vi "Configure Session.vi"(8 "error in":errorcluster, 11 "Plugin in":refnum<class "Power Spectrum Density.lvclass">) -> (0 "error out":errorcluster, 3 "Plugin out":refnum<class "Power Spectrum Density.lvclass">)   [LabVIEW 2023, in "Power Spectrum Density.lvlib" / "Power Spectrum Density.lvclass"]
uses:
  Power Spectrum Density.lvclass
  C:/Program Files/National Instruments/LabVIEW 2023/vi.lib/FlexLogger/SDK/PluginSDK.lvlibp/PEFClasses/SDK/Plugin/Plugin.lvclass
  Power Spectrum Density Data.ctl
  <vilib>/measure/maspectr.llb/Power Spectrum and PSD Export Mode.ctl
  <vilib>/Analysis/4window.llb/windowTd.ctl
  <vilib>/FlexLogger/SDK/PluginSDK.lvlibp/PEFClasses/SDK/Processing Element/Timing Parameters.ctl
  <vilib>/FlexLogger/SDK/PluginSDK.lvlibp/PEFClasses/SDK/Processing Element/Timing Method.ctl
  <vilib>/FlexLogger/SDK/PluginSDK.lvlibp/PEFClasses/SDK/System Interface/Resampling Mode.ctl
  Buffer Manager Function.ctl
  Power Spectrum Density.lvclass/Power Spectrum Density.ctl
  Power Spectrum Density Global.vi
  <vilib>/FlexLogger/SDK/PluginSDK.lvlibp/PEFClasses/SDK/Plugin/ParameterAccess/Read Enum.vi
  <vilib>/FlexLogger/SDK/PluginSDK.lvlibp/PEFClasses/SDK/Plugin/ParameterAccess/Read Boolean.vi
  <vilib>/FlexLogger/SDK/PluginSDK.lvlibp/PEFClasses/SDK/Plugin/ParameterAccess/Read I32.vi
  <vilib>/FlexLogger/SDK/PluginSDK.lvlibp/PEFClasses/SDK/Plugin/ParameterAccess/Read DBL.vi
  <vilib>/FlexLogger/SDK/PluginSDK.lvlibp/PEFClasses/SDK/Plugin/Plugin.lvclass
  <vilib>/Utility/LVLibp/NI_PackedLibraryUtility.lvlib
  <vilib>/measure/NI_MAPro.lvlib
  <vilib>/Analysis/NI_AALPro.lvlib
  <vilib>/FlexLogger/SDK/PluginSDK.lvlibp/PEFClasses/SDK/Processing Element/Processing Element.lvclass
  <vilib>/FlexLogger/SDK/PluginSDK.lvlibp/PEFClasses/SDK/System Interface/System Interface.lvclass
  C:/Program Files/National Instruments/LabVIEW 2023/vi.lib/FlexLogger/SDK/PluginSDK.lvlibp/PEFClasses/SDK/Processing Element/Processing Element.lvclass
  C:/Users/Administrator/Documents/LabVIEW Projects/FlexLogger IO Plug-ins/Power Spectrum Density/Power Spectrum Density.lvclass
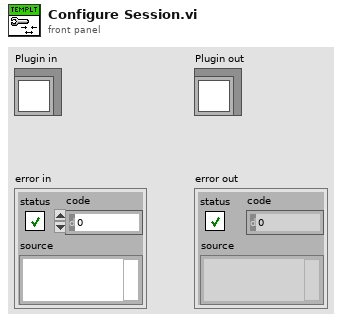
[diagram p1: front panel]
types:
  T1 = typedef "Power Spectrum Density.lvlib/Power Spectrum Density.lvclass/Buffer Manager Function.ctl" = enum16{"Get Data", "Buffer Data", "Reset Data"}
  T2 = typedef "PluginSDK.lvlibp/System Interface.lvclass/Resampling Mode.ctl" = enum16{"No Resampling", "Custom Rate", "Maximum Rate", "Minimum Rate"}
  T3 = typedef "PluginSDK.lvlibp/Processing Element.lvclass/Timing Parameters.ctl" = cluster{"Timing Method":T4, "Timing Period (ms)":i32}
  T4 = typedef "PluginSDK.lvlibp/Processing Element.lvclass/Timing Method.ctl" = enum16{"Periodic", "Immediate", "On Data Ready", "Triggered"}
  T5 = typedef "Power Spectrum Density.lvlib/Power Spectrum Density.lvclass/Power Spectrum Density Data.ctl" = cluster{"First Time":bool, "Show PSD Window":bool, "Show PSD Window Clicked":bool, "Export mode":T6, "Window":T7, "dB":bool, "Averaging parameters":cluster{"averaging mode":enum16{"No averaging", "Vector averaging", "RMS averaging", "Peak hold"}, "weighting mode":enum16{"Linear", "Exponential"}, "number of averages":u32}, "Window parameter":dbl, "Number of Samples":i32, "PSD VI Ref":refnum<vi>}
  T6 = typedef "NI_MAPro.lvlib/Power Spectrum and PSD Export Mode.ctl" = u16
  T7 = typedef "NI_AALPro.lvlib/windowTd.ctl" = u32
  T8 = enum16{"No averaging", "Vector averaging", "RMS averaging", "Peak hold"}[]
  T9 = enum16{"No averaging", "Vector averaging", "RMS averaging", "Peak hold"}
  T10 = cluster{"averaging mode":enum16{"No averaging", "Vector averaging", "RMS averaging", "Peak hold"}, "weighting mode":enum16{"Linear", "Exponential"}, u32}
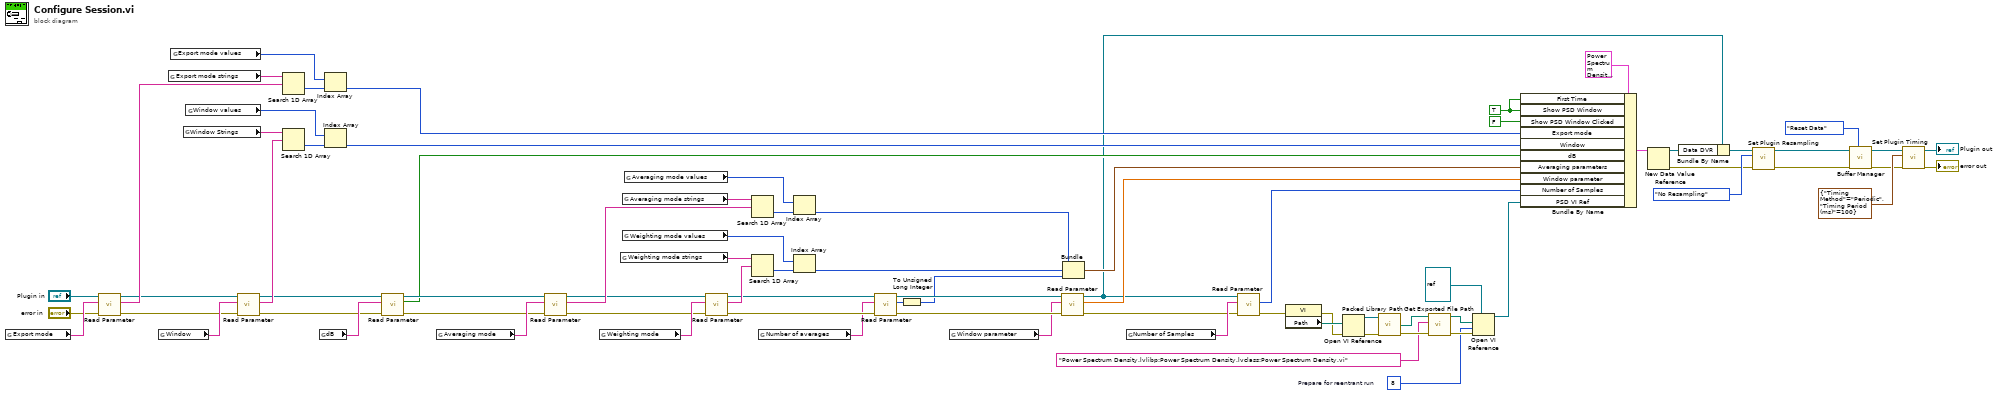
[diagram p0: block diagram]
diagram:
  w63 = 8  # Prepare for reentrant run
  w73 = TRUE ("Show Spectrogram Window")
  n1 = global read "Power Spectrum Density Global.vi" "Export mode"() -> (w59:string)
  n2 = call-poly <vilib>:"Read Parameter.vi"("error in (no error)"="error in", "Name"=w59, "Plugin in"="Plugin in") -> ("error out"=w51:errorcluster, "Value"=w77:string, "Plugin out"=w50:refnum<class "Power Spectrum Density.lvclass">)  [unwired: 4 in, 2 out]
  n3 = global read "Power Spectrum Density Global.vi" "Window"() -> (w52:string)
  n4 = global read "Power Spectrum Density Global.vi" "Export mode strings"() -> (w60:string[])
  n5 = global read "Power Spectrum Density Global.vi" "Export mode values"() -> (w61:T6[])
  n6 = global read "Power Spectrum Density Global.vi" "Window Strings"() -> (w53:string[])
  n7 = global read "Power Spectrum Density Global.vi" "Window values"() -> (w54:T7[])
  n8 = call-poly <vilib>:"Read Parameter.vi"("error in (no error)"=w51, "Name"=w52, "Plugin in"=w50) -> ("error out"=w47:errorcluster, "Value"=w56:string, "Plugin out"=w48:refnum<class "Power Spectrum Density.lvclass">)  [unwired: 4 in, 2 out]
  n9 = Search 1D Array(1D array=w60, element=w77) -> (index of element=w76:i32)  [unwired: 1 in]
  n10 = Search 1D Array(1D array=w53, element=w56) -> (index of element=w55:i32)  [unwired: 1 in]
  n11 = global read "Power Spectrum Density Global.vi" "dB"() -> (w49:string)
  n12 = Index Array(array=w61, index=w76) -> (element=w18:T6)
  n13 = Index Array(array=w54, index=w55) -> (element=w19:T7)
  n14 = call-poly <vilib>:"Read Parameter.vi"("error in (no error)"=w47, "Name"=w49, "Plugin in"=w48) -> ("error out"=w35:errorcluster, "Value"=w20:bool, "Plugin out"=w36:refnum<class "Power Spectrum Density.lvclass">)  [unwired: 5 in, 1 out]
  n15 = global read "Power Spectrum Density Global.vi" "Averaging mode"() -> (w42:string)
  n16 = call-poly <vilib>:"Read Parameter.vi"("error in (no error)"=w35, "Name"=w42, "Plugin in"=w36) -> ("error out"=w33:errorcluster, "Value"=w46:string, "Plugin out"=w34:refnum<class "Power Spectrum Density.lvclass">)  [unwired: 4 in, 2 out]
  n17 = global read "Power Spectrum Density Global.vi" "Weighting mode"() -> (w37:string)
  n18 = global read "Power Spectrum Density Global.vi" "Weighting mode strings"() -> (w38:string[])
  n19 = global read "Power Spectrum Density Global.vi" "Averaging mode strings"() -> (w43:string[])
  n20 = global read "Power Spectrum Density Global.vi" "Weighting mode values"() -> (w39:enum16{"Linear", "Exponential"}[])
  n21 = global read "Power Spectrum Density Global.vi" "Averaging mode values"() -> (w44:T8)
  n22 = call-poly <vilib>:"Read Parameter.vi"("error in (no error)"=w33, "Name"=w37, "Plugin in"=w34) -> ("error out"=w31:errorcluster, "Value"=w41:string, "Plugin out"=w32:refnum<class "Power Spectrum Density.lvclass">)  [unwired: 4 in, 2 out]
  n23 = Search 1D Array(1D array=w43, element=w46) -> (index of element=w45:i32)  [unwired: 1 in]
  n24 = Search 1D Array(1D array=w38, element=w41) -> (index of element=w40:i32)  [unwired: 1 in]
  n25 = global read "Power Spectrum Density Global.vi" "Number of averages"() -> (w30:string)
  n26 = Index Array(array=w44, index=w45) -> (element=w26:T9)
  n27 = Index Array(array=w39, index=w40) -> (element=w25:enum16{"Linear", "Exponential"})
  n28 = call-poly <vilib>:"Read Parameter.vi"("error in (no error)"=w31, "Name"=w30, "Plugin in"=w32) -> ("error out"=w78:errorcluster, "Value"=w24:i32, "Plugin out"=w79:refnum<class "Power Spectrum Density.lvclass">)  [unwired: 5 in, 1 out]
  n29 = To Unsigned Long Integer(number=w24) -> (unsigned 32bit integer=w23:u32)
  n30 = global read "Power Spectrum Density Global.vi" "Window parameter"() -> (w29:string)
  n31 = call-poly <vilib>:"Read Parameter.vi"("error in (no error)"=w78, "Name"=w29, "Plugin in"=w79) -> ("error out"=w3:errorcluster, "Value"=w27:dbl, "Plugin out"=w4:refnum<class "Power Spectrum Density.lvclass">)  [unwired: 5 in, 1 out]
  n32 = Bundle("averaging mode"=w26, "weighting mode"=w25, w23) -> (w22:T10)  [unwired: 1 in]
  n33 = global read "Power Spectrum Density Global.vi" "Number of Samples"() -> (w5:string)
  n34 = call-poly <vilib>:"Read Parameter.vi"("error in (no error)"=w3, "Name"=w5, "Plugin in"=w4) -> ("error out"=w2:errorcluster, "Value"=w1:i32)  [unwired: 5 in, 2 out]
  n35 = property class="VI"(error in=w2) -> (error out=w66:errorcluster, "Path"=w72:path)  [unwired: 1 in, 1 out]
  n36 = Open VI Reference(vi path=w72, error in (no error)=w66) -> (vi reference=w71:refnum<vi>, error out=w70:errorcluster)  [unwired: 4 in]
  n37 = call <vilib>:"Packed Library Path.vi"("error in (no error)"=w70, "vi reference"=w71) -> ("error out"=w68:errorcluster, "packed library path"=w69:path)  [unwired: 1 in, 1 out]
  n38 = call <vilib>:"Get Exported File Path.vi"("error in (no error)"=w68, "qualified name"="Power Spectrum Density.lvlibp:Power Spectrum Density.lvclass:Power Spectrum Density.vi", "packed library path"=w69) -> ("error out"=w64:errorcluster, "path"=w65:path)  [unwired: 7 in]
  n39 = Open VI Reference(type specifier VI Refnum (for type only)=refnum<vi> refnum, vi path=w65, options=w63, error in (no error)=w64) -> (vi reference=w6:refnum<vi>)  [unwired: 2 in, 1 out]
  n40 = Bundle By Name(cluster=T5 {"First Time"=FALSE, "Show PSD Window"=FALSE, "Show PSD Window Clicked"=FALSE, "Export mode"=0, "Window"=0, "dB"=FALSE, "Averaging parameters"={"averaging mode"=enum."No averaging", "weighting mode"=enum."Linear", "number of averages"=0}, "Window parameter"=0.0, "Number of Samples"=0, "PSD VI Ref"=refnum} ("Data"), "First Time"=w73, "Show PSD Window"=w73, "Show PSD Window Clicked"=FALSE ("Show Spectrogram Window"), "Export mode"=w18, "Window"=w19, "dB"=w20, "Averaging parameters"=w22, "Window parameter"=w27, "Number of Samples"=w1, "PSD VI Ref"=w6) -> (w74:T5)
  n41 = New Data Value Reference(data value=w74) -> (data value reference=w21:refnum<data-value>, error out=w12:errorcluster)  [unwired: 1 in]
  n42 = Bundle By Name(cluster=w4, "Data DVR"=w21) -> (w14:refnum<class "Power Spectrum Density.lvclass">)
  n43 = call <vilib>:"Set Plugin Resampling.vi"("Plugin in"=w14, "Resampling Mode"=Resampling_Mode."No Resampling", "error in (no error)"=w12) -> ("Plugin out"=w11:refnum<class "Power Spectrum Density.lvclass">, "error out"=w10:errorcluster)  [unwired: 11 in]
  n44 = call-dynamic "Buffer Manager.vi"("Function"=Buffer_Manager_Function."Reset Data", "error in"=w10, "Plugin in"=w11) -> ("error out"=w9:errorcluster, "Plugin out"=w7:refnum<class "Power Spectrum Density.lvclass">)  [unwired: 4 in, 3 out]
  n45 = call <vilib>:"Set Plugin Timing.vi"("error in (no error)"=w9, "Timing Parameters"=T3 {"Timing Method"=enum."Periodic", "Timing Period (ms)"=100}, "Plugin in"=w7) -> ("error out"=→"error out":errorcluster, "Plugin out"=→"Plugin out":refnum<class "Power Spectrum Density.lvclass">)  [unwired: 7 in]
